vi "Unreserve Sessions.vi"(8 "error in":errorcluster, 11 "session reservation in":refnum<class "Session Reservation.lvclass">) -> (0 "error out":errorcluster)   [LabVIEW 2020, in "MeasurementLink Session Management.lvlib" / "Session Reservation.lvclass"]
doc: "Unreserves all sessions. Once this VI is called, the session reservation refnum is no longer valid."
uses:
  Session Reservation.lvclass
  Session Reservation.lvclass/Session Reservation.ctl
  MeasurementLink gRPC Utilities/gRPC Client Pool/FGV Action.ctl
  MeasurementLink Session Management Client/RPC Messages/ni_measurementlink_sessionmanagement_v1_UnreserveSessionsRequest.ctl
  MeasurementLink Session Management Client/RPC Messages/ni_measurementlink_sessionmanagement_v1_SessionInformation.ctl
  MeasurementLink Session Management Client/RPC Messages/nidevice_grpc_Session.ctl
  MeasurementLink Session Management Client/RPC Messages/ni_measurementlink_sessionmanagement_v1_ChannelMapping.ctl
  MeasurementLink Measurement Server/Helpers/Error Strings Global Internal.vi
  IReservationObserver/IReservationObserver.lvclass
  MeasurementLink gRPC Utilities/gRPC Client Pool/gRPC Client Pool.lvclass
  MeasurementLink Session Management Client/MeasurementLink Session Management Client.lvlib
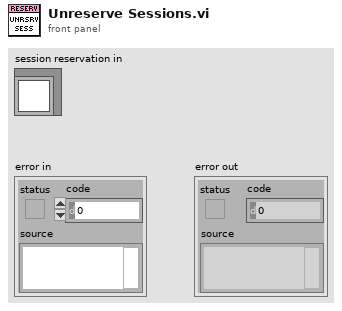
[diagram p1: front panel]
types:
  T1 = typedef "MeasurementLink Session Management Client.lvlib/ni_measurementlink_sessionmanagement_v1_UnreserveSessionsRequest.ctl" = cluster{"sessions":T2[]}
  T2 = typedef "MeasurementLink Session Management Client.lvlib/ni_measurementlink_sessionmanagement_v1_SessionInformation.ctl" = cluster{"session":T3, "resource_name":string, "channel_list":string, "instrument_type_id":string, "session_exists":bool, "channel_mappings":T4[]}
  T3 = typedef "MeasurementLink Session Management Client.lvlib/nidevice_grpc_Session.ctl" = cluster{"name":string}
  T4 = typedef "MeasurementLink Session Management Client.lvlib/ni_measurementlink_sessionmanagement_v1_ChannelMapping.ctl" = cluster{"pin_or_relay_name":string, "site":i32, "channel":string}
  T5 = typedef "MeasurementLink gRPC Utilities.lvlib/gRPC Client Pool.lvclass/FGV Action.ctl" = enum16{"Get Discovery Client", "Get Session Client", "Get Pinmap Client", "Destroy Clients"}
  T6 = typedef "MeasurementLink Session Management.lvlib/Session Reservation.lvclass/Data.ctl" = cluster{"session and driver infos":T7[], "pin or relay names":string[], "connection map":refnum<class "Connection Map.lvclass">, "pin map context":T8, "reservation observer":refnum<class "IReservationObserver.lvclass">, "dvr valid":bool}
  T7 = typedef "MeasurementLink Session Management.lvlib/Session Reservation.lvclass/Session and Driver Info.ctl" = cluster{"session info":T2, "session":variant, "instrument":refnum<class "IInstrument.lvclass">}
  T8 = typedef "MeasurementLink Session Management Client.lvlib/ni_measurementlink_PinMapContext.ctl" = cluster{"pin_map_id":string, "sites":i32[]}
  T9 = typedef "grpc-lvsupport-release.lvlib/grpcId.ctl" = u64
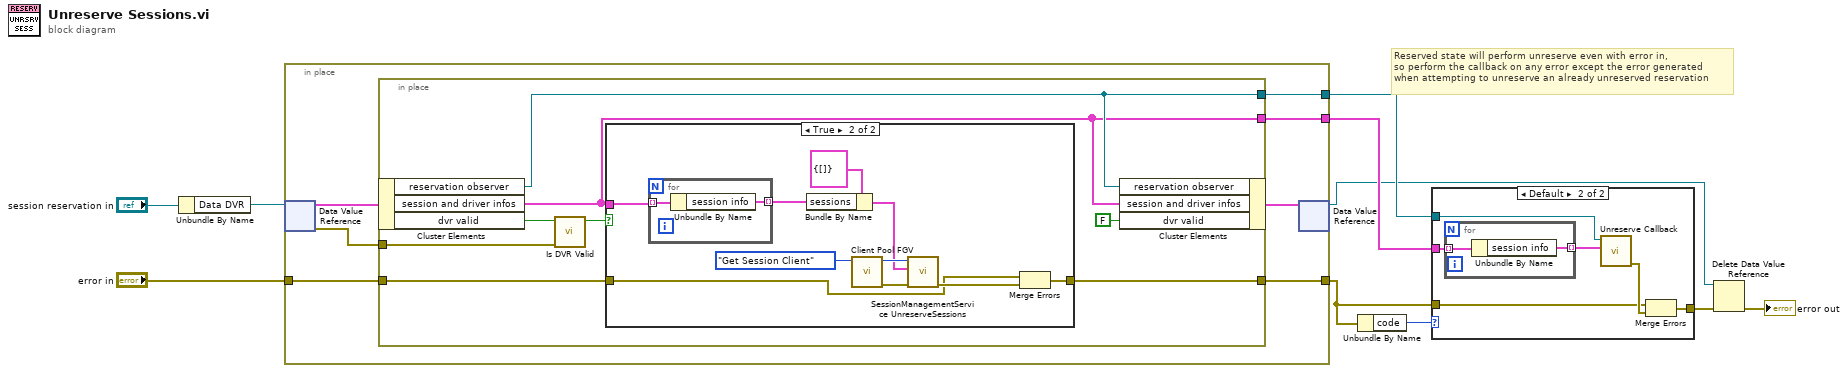
[diagram p0: block diagram]
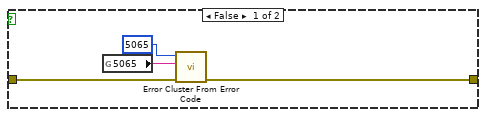
[diagram p2: hidden frame]
diagram:
  # "Reserved state will perform unreserve even with error in,\nso perform the callback on any error except the error generated\nwhen attempting to unreserve an already unreserved reservation"
  n1 = Unbundle By Name("session reservation in") -> ("Data DVR"=w8:refnum<data-value>)
  n2 = in-place {
    in-place-border: "error in" -> [w16]
    in-place-border: [w17] -> w4
    in-place-border: [w15] -> w7
    in-place-border: [w14] -> w5
    n3 = in-place-dvr #1(w8) -> (w13:T6, w11:errorcluster)
    n4 = in-place {
      in-place-border: [w18] -> w17
      in-place-border: w16 -> [w25]
      in-place-border: w11 -> [w24]
      in-place-border: [w20] -> w15
      in-place-border: [w19] -> w14
      n5 = in-place-cluster #2(w13) -> ("reservation observer"=w20:refnum<class "IReservationObserver.lvclass">, "session and driver infos"=w19:T7[], "dvr valid"=w22:bool)
      n6 = call "Is DVR Valid.vi"("dvr error in"=w24, "dvr valid"=w22) -> ("dvr valid"=w23:bool)  [unwired: 9 in]
      n7 = case shown="True" w23 {
        tunnel: w19 -> [_ w30]
        tunnel: [w26 w32] -> w18
        tunnel: w25 -> [w27 w31]
        frame False {
          n8 = global read "Error Strings Global Internal.vi" "5065"() -> (w29:string)
          n9 = call <vilib>:"Error Cluster From Error Code.vi"("error in (no error)"=w27, "error message (\"\")"=w29, "error code (0)"=5065) -> ("error out"=w26:errorcluster)  [unwired: 6 in]
        }
        frame True {
          n10 = for {
            tunnel: w30 -> [w41] mode=indexing
            tunnel: [w40] -> w34 mode=indexing
            n11 = Unbundle By Name(w41) -> ("session info"=w40:T2)
          }
          n12 = Bundle By Name(cluster=T1 {"sessions"=[]} ("Request Data"), "sessions"=w34) -> (w33:T1)
          n13 = call "Client Pool FGV.vi"("Action"=FGV_Action."Get Session Client") -> ("error out"=w37:errorcluster, "grpc client id"=w36:T9)  [unwired: 9 in]
          n14 = call "SessionManagementService UnreserveSessions.vi"("error in"=w37, "Request Data"=w33, "gRPC ID"=w36) -> ("error out"=w39:errorcluster)  [unwired: 6 in, 2 out]
          n15 = Merge Errors(w31, w39) -> (w32:errorcluster)
        }
      }
      n16 = in-place-cluster #2("reservation observer"=w20, "session and driver infos"=w19, "dvr valid"=FALSE) -> (w12:T6)
    }
    n17 = in-place-dvr #1(w12) -> (w1:refnum<data-value>)  [unwired: 1 out]
  }
  n18 = Unbundle By Name(w4) -> ("code"=w6:i32)
  n19 = case shown="Default" w6 {
    tunnel: w4 -> [w42 w43]
    tunnel: [w42 w44] -> w3
    tunnel: w5 -> [_ w46]
    tunnel: w7 -> [_ w45]
    frame 5065 {
    }
    frame Default {
      n20 = for {
        tunnel: w46 -> [w50] mode=indexing
        tunnel: [w49] -> w48 mode=indexing
        n21 = Unbundle By Name(w50) -> ("session info"=w49:T2)
      }
      n22 = call-dynamic "Unreserve Callback.vi"("session infos"=w48, "reservation observer in"=w45) -> ("error out"=w47:errorcluster)  [unwired: 8 in, 1 out]
      n23 = Merge Errors(w43, w47) -> (w44:errorcluster)
    }
  }
  n24 = Delete Data Value Reference(data value reference=w1, error in=w3) -> (error out=→"error out":errorcluster)  [unwired: 1 out]
